vi "Func1.vi"(8 "error in (no error)":errorcluster, 11 "Subject in":refnum<class "Subject.lvclass">) -> (0 "error out":errorcluster, 3 "Subject out":refnum<class "Subject.lvclass">)   [LabVIEW 2014, in "Normal Proxy.lvlib" / "Subject.lvclass"]
uses:
  Subject.lvclass
  Subject.lvclass/Subject.ctl
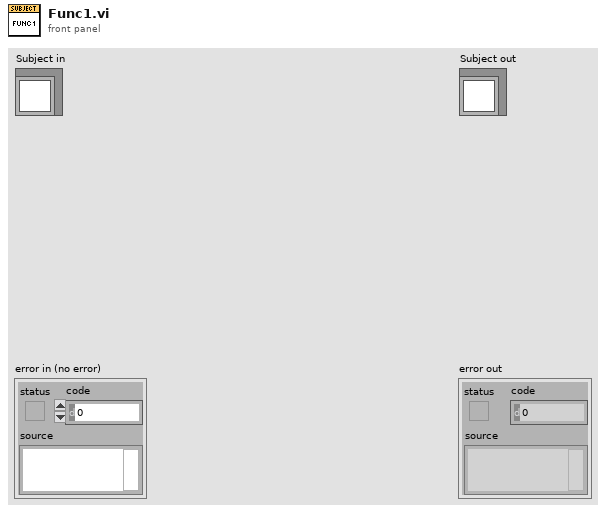
[diagram p1: front panel]
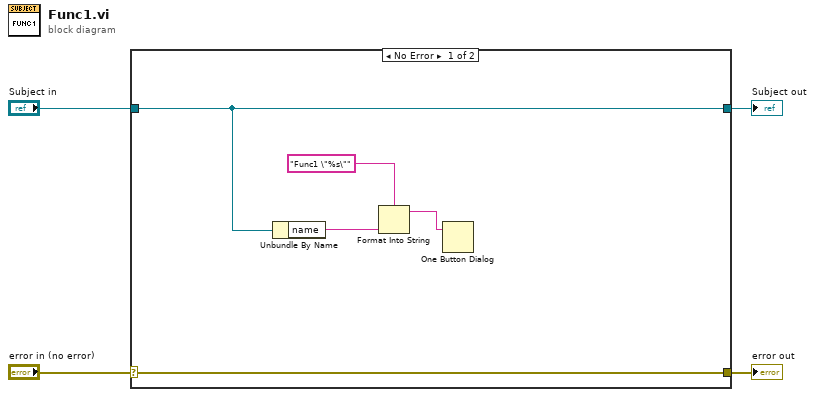
[diagram p0: block diagram]
diagram:
  n1 = case shown="No Error" "error in (no error)" {
    selector: "error in (no error)" -> [w9 w11]
    tunnel: [w9 w11] -> w3
    tunnel: [w8 w10] -> w1
    tunnel: "Subject in" -> [w8 w10]
    frame No Error {
      n2 = Unbundle By Name(w8) -> ("name"=w7:string)
      n3 = Format Into String(format string="Func1 \"%s\"", w7) -> (resulting string=w5:string)  [unwired: 2 in, 1 out]
      n4 = One Button Dialog(message=w5) -> ()  [unwired: 1 in, 1 out]
    }
    frame Error {
    }
  }
  "error out" <- w3
  "Subject out" <- w1
